vi "Build DashBoard Data.vi"(11 "Dashboard Enables":T3={"Analog Module 1"=[TRUE, TRUE, TRUE, TRUE, TRUE, TRUE, TRUE, TRUE], "Analog Module 2"=[FALSE, FALSE, FALSE, FALSE, FALSE, FALSE, FALSE, FALSE], "Digital Module 1"=TRUE, "Digital Module 2"=FALSE, "Solenoid Module"=TRUE}) -> ()   [LabVIEW 2011]
doc: "This VI builds data and sends it back to the dashboard PC program. By default it sends back the raw values for the first analog, digital, and solenoid module. Modify it to send back the data you want to view. Consider adding higher level data to the Dashboard Datatype.ctl and to this VI. Then update the Dashboard to display the data however you like.\n\nThis software is licensed. Open the labview\\readme\\WPI Robotics Library Open Source License.txt file for more information."
uses:
  DashboardEnable.ctl
  Dashboard Datatype.ctl
  <vilib>/Rock Robotics/WPI/DriverStation/WPI_DriverStationDigitalData.ctl
  Robot Global Data.vi
panel:
  out "Dashboard Data":T1
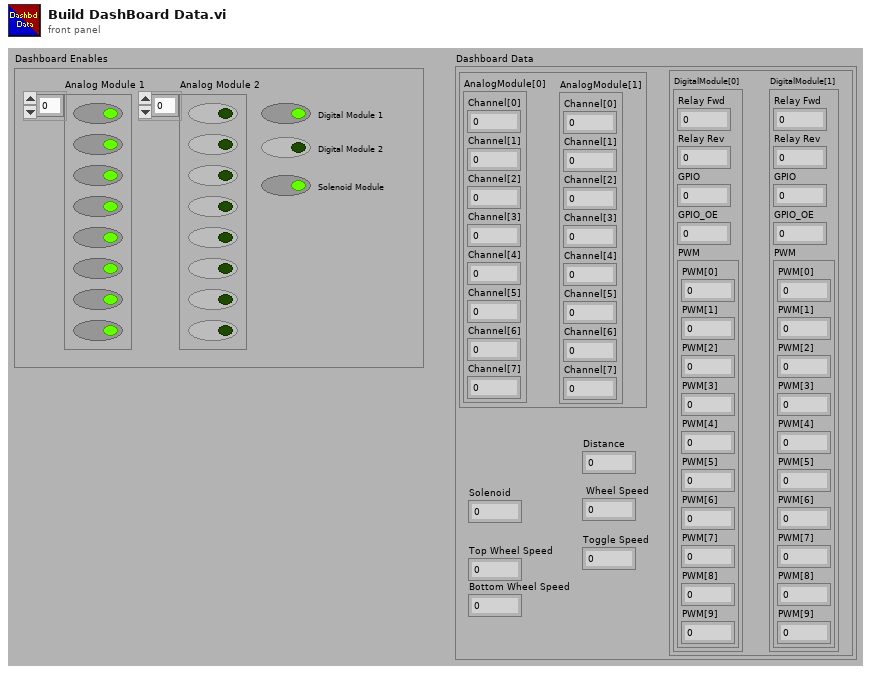
[diagram p1: front panel]
types:
  T1 = typedef "Dashboard Datatype.ctl" = cluster{cluster{"AnalogModule[0]":cluster{"Channel[0]":sgl, "Channel[1]":sgl, "Channel[2]":sgl, "Channel[3]":sgl, "Channel[4]":sgl, "Channel[5]":sgl, "Channel[6]":sgl, "Channel[7]":sgl}, "AnalogModule[1]":cluster{"Channel[0]":sgl, "Channel[1]":sgl, "Channel[2]":sgl, "Channel[3]":sgl, "Channel[4]":sgl, "Channel[5]":sgl, "Channel[6]":sgl, "Channel[7]":sgl}}, cluster{"DigitalModule[0]":T2, "DigitalModule[1]":T2}, "Solenoid":u8, " Wheel Speed":dbl, "Toggle Speed":dbl, "Distance":dbl, "Top Wheel Speed":dbl, "Bottom Wheel Speed":dbl}
  T2 = typedef "WPI_DriverStationDigitalData.ctl" = cluster{"Relay Fwd":u8, "Relay Rev":u8, "GPIO":u16, "GPIO_OE":u16, "PWM":cluster{"PWM[0]":u8, "PWM[1]":u8, "PWM[2]":u8, "PWM[3]":u8, "PWM[4]":u8, "PWM[5]":u8, "PWM[6]":u8, "PWM[7]":u8, "PWM[8]":u8, "PWM[9]":u8}}
  T3 = typedef "DashboardEnable.ctl" = cluster{"Analog Module 1":bool[], "Analog Module 2":bool[], "Digital Module 1":bool, "Digital Module 2":bool, "Solenoid Module":bool}
  T4 = cluster{"AnalogModule[0]":cluster{"Channel[0]":sgl, "Channel[1]":sgl, "Channel[2]":sgl, "Channel[3]":sgl, "Channel[4]":sgl, "Channel[5]":sgl, "Channel[6]":sgl, "Channel[7]":sgl}, "AnalogModule[1]":cluster{"Channel[0]":sgl, "Channel[1]":sgl, "Channel[2]":sgl, "Channel[3]":sgl, "Channel[4]":sgl, "Channel[5]":sgl, "Channel[6]":sgl, "Channel[7]":sgl}}
  T5 = cluster{"Channel[0]":sgl, "Channel[1]":sgl, "Channel[2]":sgl, "Channel[3]":sgl, "Channel[4]":sgl, "Channel[5]":sgl, "Channel[6]":sgl, "Channel[7]":sgl}[]
  T6 = cluster{"Channel[0]":sgl, "Channel[1]":sgl, "Channel[2]":sgl, "Channel[3]":sgl, "Channel[4]":sgl, "Channel[5]":sgl, "Channel[6]":sgl, "Channel[7]":sgl}
  T7 = cluster{"AnalogModule[0][0]":sgl, "AnalogModule[0][1]":sgl, "AnalogModule[0][2]":sgl, "AnalogModule[0][3]":sgl, "AnalogModule[0][4]":sgl, "AnalogModule[0][5]":sgl, "AnalogModule[0][6]":sgl, "AnalogModule[0][7]":sgl}
  T8 = cluster{"[0]":cluster{"Channel[0]":sgl, "Channel[1]":sgl, "Channel[2]":sgl, "Channel[3]":sgl, "Channel[4]":sgl, "Channel[5]":sgl, "Channel[6]":sgl, "Channel[7]":sgl}, "[1]":cluster{"Channel[0]":sgl, "Channel[1]":sgl, "Channel[2]":sgl, "Channel[3]":sgl, "Channel[4]":sgl, "Channel[5]":sgl, "Channel[6]":sgl, "Channel[7]":sgl}}
  T9 = cluster{"DigitalModule[0]":T2, "DigitalModule[1]":T2}
  T10 = typedef "FPGA_DIODevRef.ctl" = cluster{"DevStatus":errorcluster, "Module":T11}
  T11 = typedef "FPGA_TypedefDigitalModule.ctl" = enum16{"Digital Module 1", "Digital Module 2"}
  T12 = cluster{"[0]":u8, "[1]":u8, "[2]":u8, "[3]":u8, "[4]":u8, "[5]":u8, "[6]":u8, "[7]":u8, "[8]":u8, "[9]":u8}
  T13 = typedef "FPGA_SolenoidDevRef.ctl" = cluster{"DevStatus":errorcluster, "Module":T14}
  T14 = typedef "FPGA_TypedefSolenoidModule.ctl" = enum16{"Solenoid Module 1", "Solenoid Module 2"}
  T15 = cluster{"Set Wheel Speed":dbl, "Set Toggle Speed":dbl, "Distance Global":dbl, "Top Wheel Speed":dbl, "Bottom Wheel Speed":dbl}
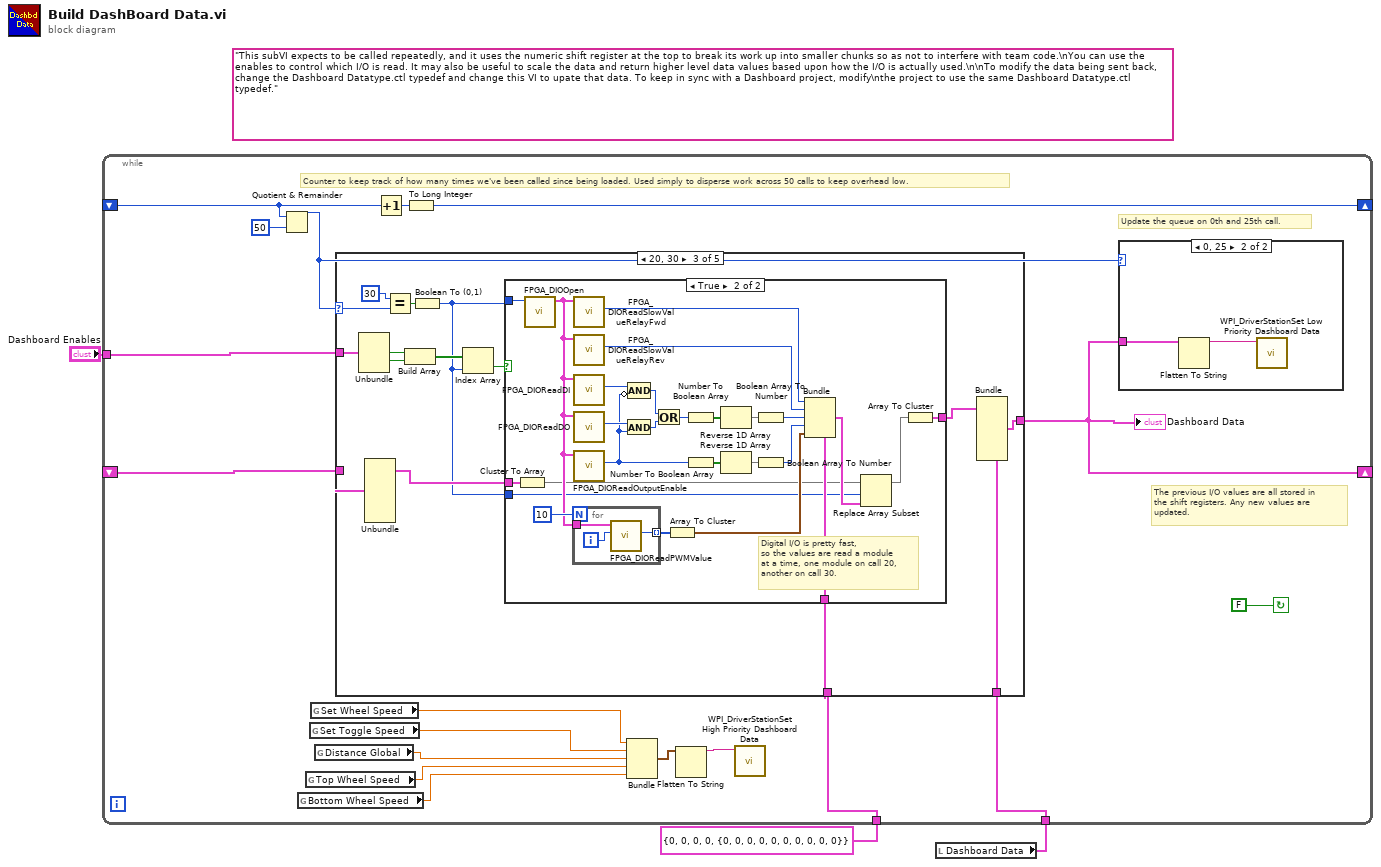
[diagram p0: block diagram]
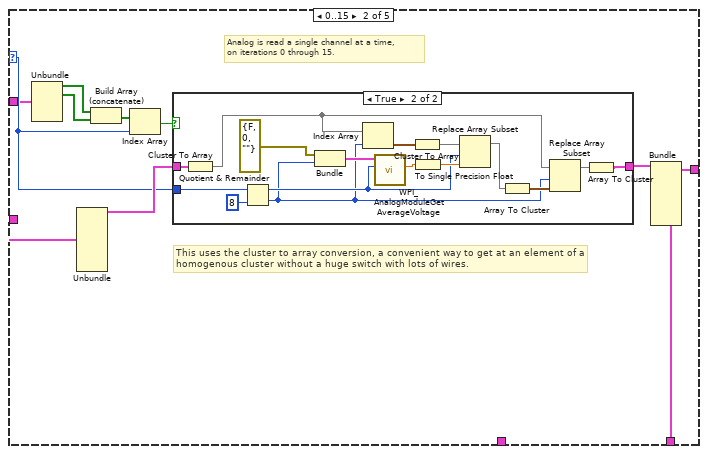
[diagram p4: hidden frame]
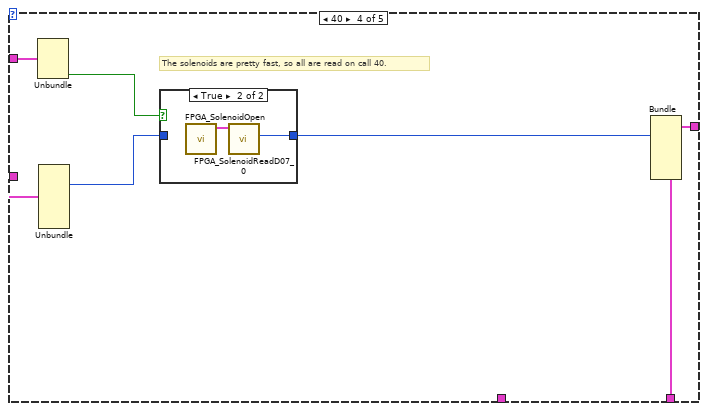
[diagram p7: hidden frame]
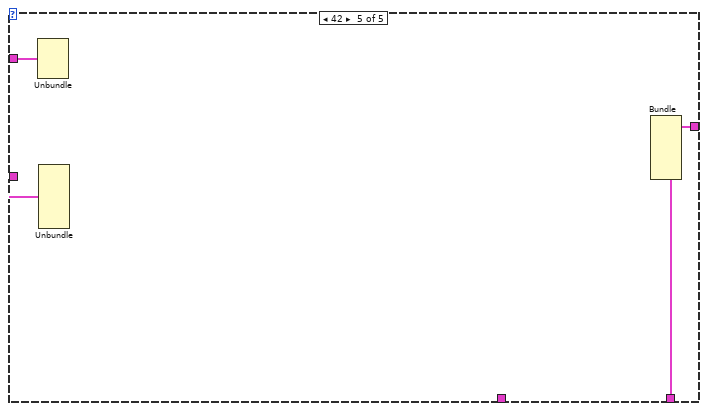
[diagram p9: hidden frame]
diagram:
  (unwired) "This subVI expects to be called repeatedly, and it uses the numeric shift register at the top to break its work up into smaller chunks so as not to interfere with team code.\nYou can use the enables to control which I/O is read. It may also be useful to scale the data and return higher level data values based upon how the I/O is actually used.\n\nTo modify the data being sent back, change the Dashboard Datatype.ctl typedef and change this VI to upate that data. To keep in sync with a Dashboard project, modify\nthe project to use the same Dashboard Datatype.ctl typedef."
  n1 = local read "Dashboard Data"() -> (w2:T1)
  n2 = while {
    shift-right: [w14] -> _
    shift-left: _ -> [w16]
    shift-right: [w11] -> _
    shift-left: _ -> [w19]
    tunnel: T2 {"Relay Fwd"=0, "Relay Rev"=0, "GPIO"=0, "GPIO_OE"=0, "PWM"={"PWM[0]"=0, "PWM[1]"=0, "PWM[2]"=0, "PWM[3]"=0, "PWM[4]"=0, "PWM[5]"=0, "PWM[6]"=0, "PWM[7]"=0, "PWM[8]"=0, "PWM[9]"=0}} ("DigitalModule[1]") -> [w18]
    tunnel: w2 -> [w13]
    tunnel: "Dashboard Enables" -> [w12]
    stop <- FALSE continue-if-true
    # "Counter to keep track of how many times we've been called since being loaded. Used simply to disperse work across 50 calls to keep overhead low."
    # "Update the queue on 0th and 25th call."
    # "The previous I/O values are all stored in\nthe shift registers. Any new values are\nupdated."
    n3 = Quotient & Remainder(x=w16, y=50) -> (x-y*floor(x/y)=w15:i32)  [unwired: 1 out]
    n4 = global read "Robot Global Data.vi" "Bottom Wheel Speed"() -> (w4:dbl)
    n5 = global read "Robot Global Data.vi" "Top Wheel Speed"() -> (w5:dbl)
    n6 = global read "Robot Global Data.vi" "Set Toggle Speed"() -> (w9:dbl)
    n7 = global read "Robot Global Data.vi" "Set Wheel Speed"() -> (w10:dbl)
    n8 = global read "Robot Global Data.vi" "Distance Global"() -> (w8:dbl)
    n9 = case shown="20, 30" w15 {
      selector: w15 -> [_ w30 w63 _ _]
      tunnel: [w24 w26 w54 w101 w109] -> w11
      tunnel: w19 -> [w24 w25 w56 w103 w110]
      tunnel: w18 -> [_ _ w67 _ _]
      tunnel: w13 -> [_ w32 w55 w100 w108]
      tunnel: w12 -> [_ w29 w61 w104 w111]
      frame Default {
        # "Don't update any I/O"
      }
      frame 0..15 {
        # "This uses the cluster to array conversion, a convenient way to get at an element of a\nhomogenous cluster without a huge switch with lots of wires."
        # "Analog is read a single channel at a time,\non iterations 0 through 15."
        n10 = Unbundle(w29) -> ("Analog Module 1"=w28:bool[], "Analog Module 2"=w27:bool[])  [unwired: 3 out]
        n11 = Unbundle(w25) -> (w31:T4)  [unwired: 7 out]
        n12 = Build Array (concatenate)(w28, w27) -> (w34:bool[])
        n13 = Index Array(array=w34, index=w30) -> (element=w35:bool)
        n14 = case shown="True" w35 {
          tunnel: w30 -> [_ w43]
          tunnel: [w36 w40] -> w33
          tunnel: w31 -> [w36 w39]
          frame False {
          }
          frame True {
            n15 = Cluster To Array(cluster=w39) -> (array=w38:T5)
            n16 = Quotient & Remainder(x=w43, y=8) -> (x-y*floor(x/y)=w42:i32, floor(x/y)=w37:i32)
            n17 = Bundle("DevStatus"=errorcluster {"status"=FALSE, "code"=0, "source"=""}, w37) -> (w51:cluster{"DevStatus":errorcluster, i32})  [unwired: 1 out]
            n18 = Index Array(array=w38, index=w37) -> (element=w45:T6)
            n19 = call <vilib>:"WPI_AnalogModuleGetAverageVoltage.vi"("Channel"=w42, "AnalogModuleDevStatus"=w51) -> ("Average Voltage"=w48:dbl)  [unwired: 1 in, 8 out]
            n20 = Cluster To Array(cluster=w45) -> (array=w44:sgl[])
            n21 = To Single Precision Float(number=w48) -> (single precision float=w47:sgl)
            n22 = Replace Array Subset(array=w44, new element=w47, index=w42) -> (w46:sgl[])
            n23 = Array To Cluster(array=w46) -> (cluster=w50:T7)
            n24 = Replace Array Subset(array=w38, new element=w50, index=w37) -> (w41:T5)
            n25 = Array To Cluster(array=w41) -> (cluster=w40:T8)
          }
        }
        n26 = Bundle(cluster=w32, w33) -> (w26:T1)  [unwired: 7 out]
      }
      frame 20, 30 {
        n27 = Unbundle(w61) -> ("Digital Module 1"=w60:bool, "Digital Module 2"=w59:bool)  [unwired: 3 out]
        n28 = Unbundle(w56) -> (w58:T9)  [unwired: 7 out]
        n29 = Equal?(x=30, y=w63) -> (x = y?=w65:bool)
        n30 = Build Array(w60, w59) -> (w62:bool[])
        n31 = Boolean To (0,1)(Boolean=w65) -> (0, 1=w53:i16)
        n32 = Index Array(array=w62, index=w53) -> (element=w64:bool)
        n33 = case shown="True" w64 {
          tunnel: w67 -> [_ w76]
          tunnel: [w68 w69] -> w57
          tunnel: w53 -> [_ w74]
          tunnel: w53 -> [_ w73]
          tunnel: w58 -> [w68 w72]
          frame False {
          }
          frame True {
            # "Digital I/O is pretty fast,\nso the values are read a module\nat a time, one module on call 20,\nanother on call 30."
            n34 = Cluster To Array(cluster=w72) -> (array=w71:T2[])
            n35 = call <vilib>:"FPGA_DIOOpen.vi"("Module (Module 1)"=w74) -> ("DIODeviceRef"=w92:T10)  [unwired: 1 in, 9 out]
            n36 = for {
              N: 10 -> [_]
              tunnel: w92 -> [w97]
              tunnel: [w95] -> w93 mode=indexing
              i -> [w96]
              n37 = call <vilib>:"FPGA_DIOReadPWMValue.vi"("PWMChannel"=w96, "DIODeviceRef In"=w97) -> ("PWMValue"=w95:u8)  [unwired: 1 in, 8 out]
            }
            n38 = call <vilib>:"FPGA_DIOReadSlowValueRelayFwd.vi"("DIODeviceRef In"=w92) -> ("Relay Forward"=w85:u8)  [unwired: 1 in, 9 out]
            n39 = call <vilib>:"FPGA_DIOReadSlowValueRelayRev.vi"("DIODeviceRef In"=w92) -> ("Relay Reverse"=w86:u8)  [unwired: 1 in, 9 out]
            n40 = call <vilib>:"FPGA_DIOReadDI.vi"("DIODeviceRef In"=w92) -> ("DI"=w90:u16)  [unwired: 1 in, 9 out]
            n41 = call <vilib>:"FPGA_DIOReadDO.vi"("DIODeviceRef In"=w92) -> ("DO"=w89:u16)  [unwired: 1 in, 9 out]
            n42 = call <vilib>:"FPGA_DIOReadOutputEnable.vi"("DIODeviceRef In"=w92) -> ("OutputEnable"=w80:u16)  [unwired: 1 in, 9 out]
            n43 = And(x=w89, y=w80) -> (x .and. y?=w88:u16)
            n44 = Compound Arithmetic op=AND(w90, invert w80) -> (w87:u16)
            n45 = Or(x=w87, y=w88) -> (x .or. y?=w78:u16)
            n46 = Array To Cluster(array=w93) -> (cluster=w91:T12)
            n47 = Number To Boolean Array(number=w78) -> (Boolean array=w83:bool[])
            n48 = Number To Boolean Array(number=w80) -> (Boolean array=w82:bool[])
            n49 = Reverse 1D Array(array=w83) -> (reversed array=w84:bool[])
            n50 = Reverse 1D Array(array=w82) -> (reversed array=w81:bool[])
            n51 = Boolean Array To Number(Boolean array=w84) -> (number=w77:u32)
            n52 = Boolean Array To Number(Boolean array=w81) -> (number=w79:u32)
            n53 = Bundle(cluster=w76, "Relay Fwd"=w85, "Relay Rev"=w86, "GPIO"=w77, "GPIO_OE"=w79, "PWM"=w91) -> (w75:T2)
            n54 = Replace Array Subset(array=w71, new element=w75, index=w73) -> (w70:T2[])
            n55 = Array To Cluster(array=w70) -> (cluster=w69:cluster{"[0]":T2, "[1]":T2})
          }
        }
        n56 = Bundle(cluster=w55, w57) -> (w54:T1)  [unwired: 7 out]
      }
      frame 40 {
        # "The solenoids are pretty fast, so all are read on call 40."
        n57 = Unbundle(w104) -> ("Solenoid Module"=w98:bool)  [unwired: 4 out]
        n58 = Unbundle(w103) -> ("Solenoid"=w102:u8)  [unwired: 7 out]
        n59 = case shown="True" w98 {
          tunnel: [w105 w106] -> w99
          tunnel: w102 -> [w105 _]
          frame False {
          }
          frame True {
            n60 = call <vilib>:"FPGA_SolenoidOpen.vi"() -> ("SolenoidDevRef"=w107:T13)  [unwired: 2 in, 9 out]
            n61 = call <vilib>:"FPGA_SolenoidReadD07_0.vi"("SolenoidDevRef"=w107) -> ("DO7:0"=w106:u8)  [unwired: 1 in, 9 out]
          }
        }
        n62 = Bundle(cluster=w100, "Solenoid"=w99) -> (w101:T1)  [unwired: 7 out]
      }
      frame 42 {
        n63 = Unbundle(w111) -> ()  [unwired: 5 out]
        n64 = Unbundle(w110) -> ()  [unwired: 8 out]
        n65 = Bundle(cluster=w108) -> (w109:T1)  [unwired: 8 out]
      }
    }
    "Dashboard Data" <- w11
    n66 = Increment(x=w16) -> (x+1=w21:i32)
    n67 = To Long Integer(number=w21) -> (32bit integer=w14:i32)
    n68 = Bundle("Set Wheel Speed"=w10, "Set Toggle Speed"=w9, "Distance Global"=w8, "Top Wheel Speed"=w5, "Bottom Wheel Speed"=w4) -> (w7:T15)  [unwired: 1 in]
    n69 = Flatten To String(anything=w7) -> (data string=w6:string)  [unwired: 1 in, 4 out]
    n70 = call <vilib>:"WPI_DriverStationSet High Priority Dashboard Data.vi"("User Data"=w6) -> ()  [unwired: 10 in, 1 out]
    n71 = case shown="0, 25" w15 {
      tunnel: w11 -> [_ w23]
      frame Default {
      }
      frame 0, 25 {
        n72 = Flatten To String(anything=w23) -> (data string=w22:string)  [unwired: 1 in, 4 out]
        n73 = call <vilib>:"WPI_DriverStationSet Low Priority Dashboard Data.vi"("User Data"=w22) -> ()  [unwired: 1 in, 10 out]
      }
    }
  }
